vi "Receive Messages.vi"(6 "Wait Time":i32=-1, 8 "error in (no error)":errorcluster, 9 "Visibility Timeout":i32, 10 "Max Number of Messages":i32=1, 11 "SQS in":refnum<class "NI_AWS_SQS.lvclass">) -> (0 "error out":errorcluster, 2 "Messages":T1[](array[typedef]), 3 "SQS out":refnum<class "NI_AWS_SQS.lvclass">)   [LabVIEW 2015, in "NI_AWS_SQS.lvclass"]
uses:
  NI_AWS_SQS.lvclass
  Message.ctl
  Message Attribute Value Pair.ctl
  Message Attribute.ctl
  Core/Name Value Pair.ctl
  Core/Request Options.ctl
  NI_AWS_SQS.lvclass/NI_AWS_SQS.ctl
  Read Account Number.vi
  Read Name.vi
  Core/NI_AWS_Core.lvclass
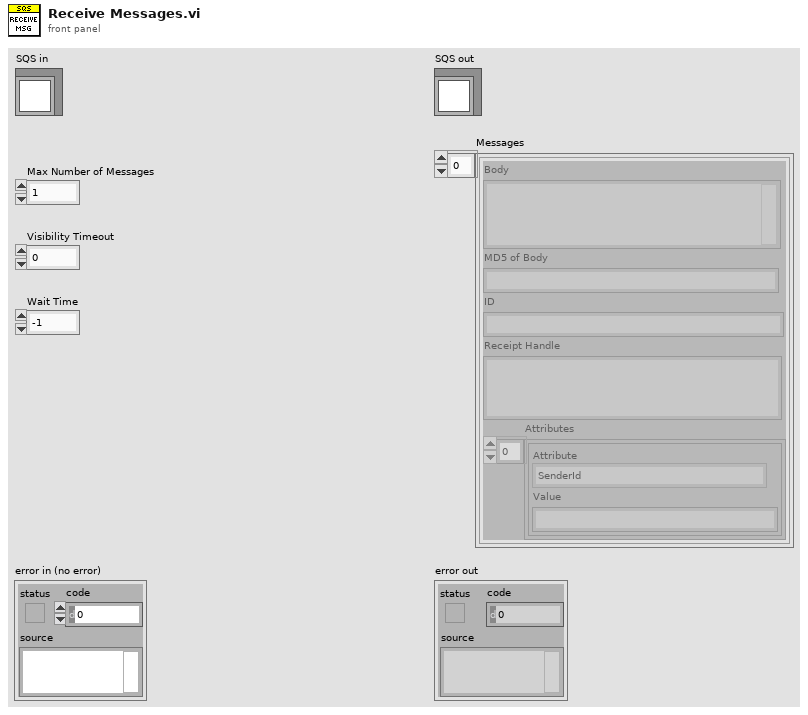
[diagram p1: front panel]
types:
  T1 = typedef "NI_AWS_SQS.lvclass/Message.ctl" = cluster{"Body":string, "MD5 of Body":string, "ID":string, "Receipt Handle":string, "Attributes":T2[]}
  T2 = typedef "NI_AWS_SQS.lvclass/Message Attribute Value Pair.ctl" = cluster{"Attribute":T3, "Value":string}
  T3 = typedef "NI_AWS_SQS.lvclass/Message Attribute.ctl" = enum16{"SenderId", "SentTimestamp", "ApproximateReceiveCount", "ApproximateFirstReceiveTimestamp"}
  T4 = typedef "NI_AWS_Core.lvclass/Name Value Pair.ctl" = cluster{"name":string, "value":string}
  T5 = typedef "NI_AWS_Core.lvclass/Request Options.ctl" = cluster{"request headers":T4[], "request parameters":T4[], "request body":string}
  T6 = typedef "NI_AWS_Core.lvclass/Response.ctl" = cluster{"Headers":string, "Body":string}
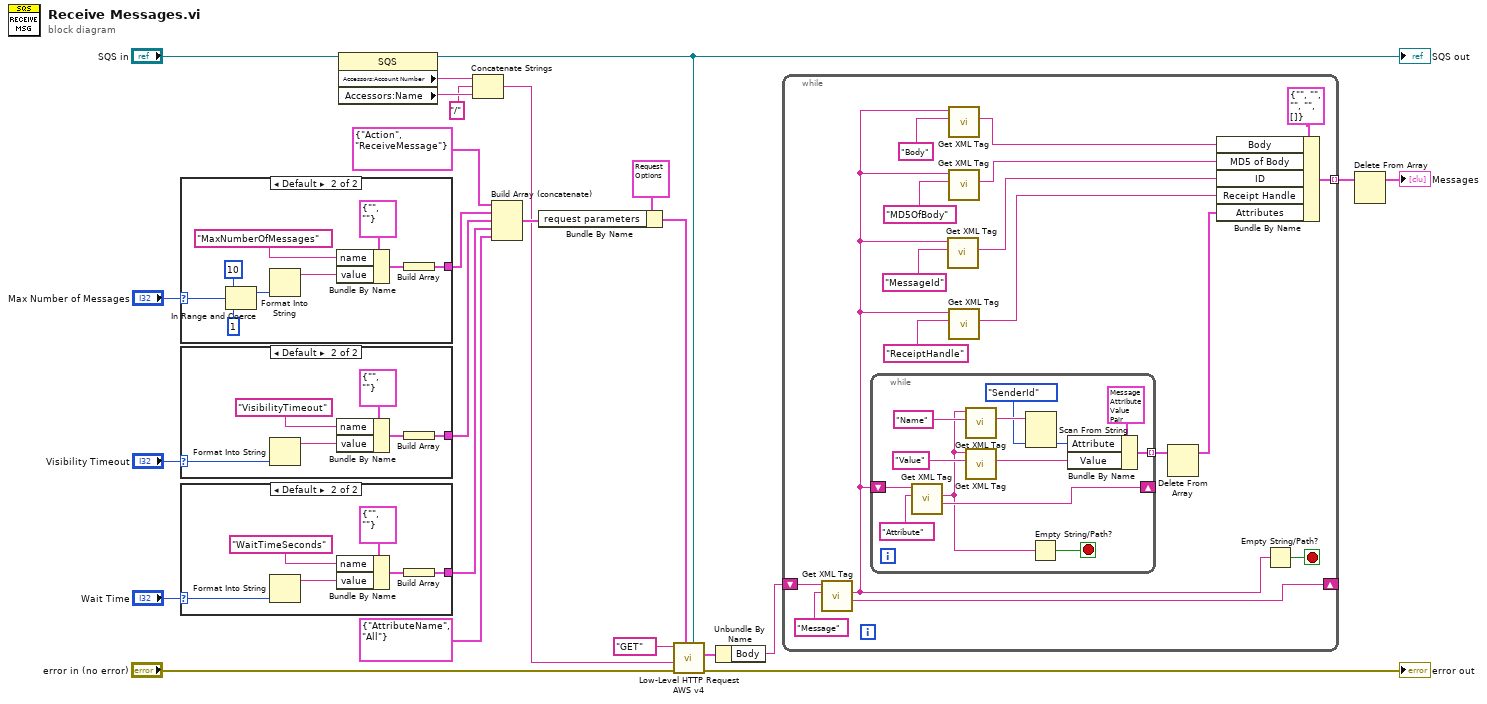
[diagram p0: block diagram]
diagram:
  n1 = case shown="Default" "Max Number of Messages" {
    selector: "Max Number of Messages" -> [_ w31]
    tunnel: [_ w25] -> w9
    frame ..1 {
    }
    frame Default {
      n2 = In Range and Coerce(upper limit=10, x=w31, lower limit=1) -> (coerced(x)=w28:i32)  [unwired: 1 out]
      n3 = Format Into String(w28) -> (resulting string=w27:string)  [unwired: 3 in, 1 out]
      n4 = Bundle By Name(cluster=T4 {"name"="", "value"=""} ("element"), "name"="MaxNumberOfMessages", "value"=w27) -> (w26:T4)
      n5 = Build Array(w26) -> (w25:T4[])
    }
  }
  n6 = case shown="Default" "Visibility Timeout" {
    selector: "Visibility Timeout" -> [_ w39]
    tunnel: [_ w34] -> w7
    frame ..0 {
    }
    frame Default {
      n7 = Format Into String(w39) -> (resulting string=w36:string)  [unwired: 3 in, 1 out]
      n8 = Bundle By Name(cluster=T4 {"name"="", "value"=""} ("element"), "name"="VisibilityTimeout", "value"=w36) -> (w35:T4)
      n9 = Build Array(w35) -> (w34:T4[])
    }
  }
  n10 = case shown="Default" "Wait Time" {
    selector: "Wait Time" -> [_ w45]
    tunnel: [_ w40] -> w5
    frame ..-1 {
    }
    frame Default {
      n11 = Format Into String(w45) -> (resulting string=w42:string)  [unwired: 3 in, 1 out]
      n12 = Bundle By Name(cluster=T4 {"name"="", "value"=""} ("element"), "name"="WaitTimeSeconds", "value"=w42) -> (w41:T4)
      n13 = Build Array(w41) -> (w40:T4[])
    }
  }
  n14 = property class="SQS"(reference="SQS in") -> (reference out=w16:refnum<class "NI_AWS_SQS.lvclass">, "Accessors:Account Number"=w15:string, "Accessors:Name"=w14:string)  [unwired: 1 in, 1 out]
  "SQS out" <- w16
  n15 = Concatenate Strings(w15, "/", w14) -> (w12:string)
  n16 = Build Array (concatenate)(T4 {"name"="Action", "value"="ReceiveMessage"} ("Cluster"), w9, w7, w5, T4 {"name"="AttributeName", "value"="All"} ("Cluster")) -> (w17:T4[])
  n17 = Bundle By Name(cluster=T5 {"request headers"=[], "request parameters"=[{"name"="Action", "value"="ListQueues"}], "request body"=""} ("Request Options"), "request parameters"=w17) -> (w18:T5)
  n18 = call "Low-Level HTTP Request AWS v4.vi"("AWS Core"=w16, "Request Options"=w18, "error in (no error)"="error in (no error)", "URL Suffix"=w12, "HTTP-Verb"="GET") -> ("error out"=→"error out":errorcluster, "Response"=w21:T6)  [unwired: 4 in, 1 out]
  n19 = Unbundle By Name(w21) -> ("Body"=w20:string)
  n20 = while {
    shift-right: [w61] -> _
    shift-left: w20 -> [w62]
    tunnel: [w56] -> w3 mode=indexing
    stop <- w60 stop-if-true
    n21 = call "Get XML Tag.vi"("Tag name"="Message", "XML String in"=w62) -> ("Remaining string"=w61:string, "Tag value"=w48:string)  [unwired: 5 in, 3 out]
    n22 = while {
      shift-right: [w74] -> _
      shift-left: w48 -> [w75]
      tunnel: [w70] -> w47 mode=indexing
      stop <- w72 stop-if-true
      n23 = call "Get XML Tag.vi"("Tag name"="Attribute", "XML String in"=w75) -> ("Remaining string"=w74:string, "Tag value"=w67:string)  [unwired: 5 in, 3 out]
      n24 = call "Get XML Tag.vi"("Tag name"="Name", "XML String in"=w67) -> ("Tag value"=w64:string)  [unwired: 5 in, 4 out]
      n25 = call "Get XML Tag.vi"("Tag name"="Value", "XML String in"=w67) -> ("Tag value"=w66:string)  [unwired: 5 in, 4 out]
      n26 = Scan From String(input string=w64, default 1=Message_Attribute."SenderId" ("Attribute")) -> (output 1=w65:T3)  [unwired: 3 in, 3 out]
      n27 = Empty String/Path?(string/path=w67) -> (empty?=w72:bool)
      n28 = Bundle By Name(cluster=T2 {"Attribute"=enum."ApproximateFirstReceiveTimestamp", "Value"=""} ("Message Attribute Value Pair"), "Attribute"=w65, "Value"=w66) -> (w70:T2)
    }
    n29 = call "Get XML Tag.vi"("Tag name"="MessageId", "XML String in"=w48) -> ("Tag value"=w52:string)  [unwired: 5 in, 4 out]
    n30 = call "Get XML Tag.vi"("Tag name"="Body", "XML String in"=w48) -> ("Tag value"=w53:string)  [unwired: 5 in, 4 out]
    n31 = call "Get XML Tag.vi"("Tag name"="MD5OfBody", "XML String in"=w48) -> ("Tag value"=w55:string)  [unwired: 5 in, 4 out]
    n32 = call "Get XML Tag.vi"("Tag name"="ReceiptHandle", "XML String in"=w48) -> ("Tag value"=w49:string)  [unwired: 5 in, 4 out]
    n33 = Delete From Array(array=w47) -> (array with subset deleted=w46:T2[])  [unwired: 2 in, 1 out]
    n34 = Bundle By Name(cluster=T1 {"Body"="", "MD5 of Body"="", "ID"="", "Receipt Handle"="", "Attributes"=[]} ("Message"), "Body"=w53, "MD5 of Body"=w55, "ID"=w52, "Receipt Handle"=w49, "Attributes"=w46) -> (w56:T1)
    n35 = Empty String/Path?(string/path=w48) -> (empty?=w60:bool)
  }
  n36 = Delete From Array(array=w3) -> (array with subset deleted=→"Messages":T1[])  [unwired: 2 in, 1 out]
